vi "readinDioXML.vi"(8 "error in (no error)":errorcluster, 10 "channel_configXML":refnum<class "NativeXML.lvclass">, 11 "deviceDataBase in":refnum<class "deviceDataBase.lvclass">) -> (0 "error out":errorcluster, 2 "device.lvclass out":refnum<class "device.lvclass">, 3 "deviceDataBase out":refnum<class "deviceDataBase.lvclass">)   [LabVIEW 2009, in "Tools.lvlib" / "DatabaseHelpers.lvlib" / "deviceDataBase.lvclass"]
uses:
  deviceDataBase.lvclass
  NativeXML/NativeXML.lvclass
  Database Objects/device/device.lvclass
  Database Objects/device/DigitalDevice/DigitalDevice.lvclass
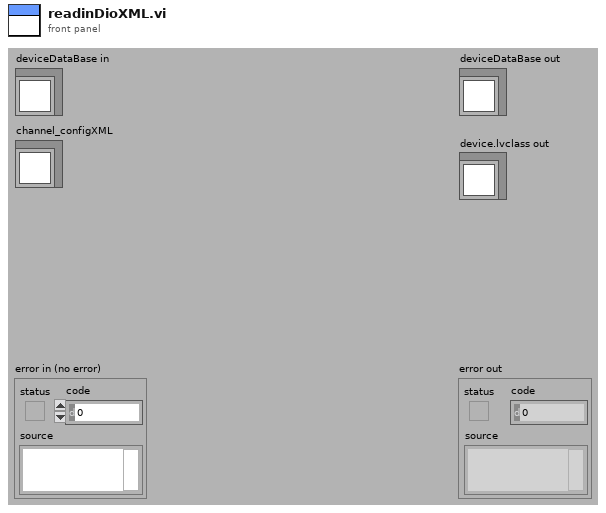
[diagram p1: front panel]
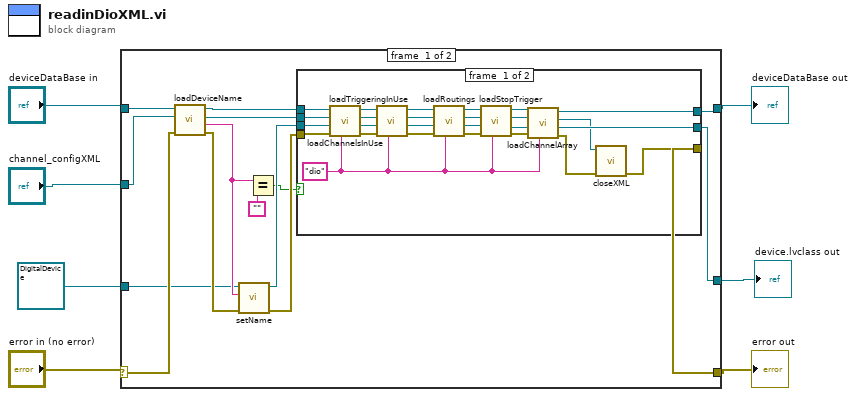
[diagram p0: block diagram]
diagram:
  n1 = case shown="No Error" "error in (no error)" {
    selector: "error in (no error)" -> [w21 w53]
    tunnel: [w9 w53] -> w3
    tunnel: [w14 w52] -> w4
    tunnel: "deviceDataBase in" -> [w22 w52]
    tunnel: "channel_configXML" -> [w20 _]
    tunnel: [w10 _] -> w2
    tunnel: refnum<class "DigitalDevice.lvclass"> refnum ("Tools.lvlib:DatabaseHelpers.lvlib:DigitalDevice.lvclass") -> [w8 _]
    frame #0 {
      n2 = call "loadDeviceName.vi"("error in (no error)"=w21, "NativeXML in"=w20, "deviceDataBase in"=w22) -> ("error out"=w19:errorcluster, "deviceName"=w12:string, "NativeXML out"=w16:refnum<class "NativeXML.lvclass">, "deviceDataBase out"=w18:refnum<class "deviceDataBase.lvclass">)  [unwired: 5 in]
      n3 = call "setName.vi"("error in (no error)"=w19, "name"=w12, "device.lvclass in"=w8) -> ("error out"=w17:errorcluster, "device.lvclass out"=w15:refnum<class "DigitalDevice.lvclass">)  [unwired: 7 in]
      n4 = Equal?(x=w12, y="") -> (x = y?=w11:bool)
      n5 = case shown="False" w11 {
        tunnel: w18 -> [w48 w51]
        tunnel: w17 -> [w47 w49]
        tunnel: w16 -> [w46 _]
        tunnel: w15 -> [w45 w50]
        tunnel: [w23 w49] -> w9
        tunnel: [w40 w50] -> w10
        tunnel: [w39 w51] -> w14
        frame #0 {
          w26 = "dio"
          n6 = call "loadChannelsInUse.vi"("type"=w26, "error in (no error)"=w47, "device.lvclass"=w45, "NativeXML in"=w46, "deviceDataBase in"=w48) -> ("error out"=w44:errorcluster, "device.lvclass out"=w41:refnum<class "device.lvclass">, "NativeXML out"=w42:refnum<class "NativeXML.lvclass">, "deviceDataBase out"=w43:refnum<class "deviceDataBase.lvclass">)  [unwired: 3 in]
          n7 = call "loadTriggeringInUse.vi"("type"=w26, "error in (no error)"=w44, "device.lvclass"=w41, "NativeXML in"=w42, "deviceDataBase in"=w43) -> ("error out"=w35:errorcluster, "device.lvclass out"=w36:refnum<class "device.lvclass">, "NativeXML out"=w37:refnum<class "NativeXML.lvclass">, "deviceDataBase out"=w38:refnum<class "deviceDataBase.lvclass">)  [unwired: 3 in]
          n8 = call "loadRoutings.vi"("type"=w26, "error in (no error)"=w35, "device.lvclass"=w36, "channel_configXML"=w37, "deviceDataBase in"=w38) -> ("error out"=w27:errorcluster, "device.lvclass out"=w31:refnum<class "device.lvclass">, "channel_configXML"=w32:refnum<class "NativeXML.lvclass">, "deviceDataBase out"=w33:refnum<class "deviceDataBase.lvclass">)  [unwired: 3 in]
          n9 = call "loadStopTrigger.vi"("type"=w26, "error in (no error)"=w27, "device.lvclass"=w31, "xml in"=w32, "deviceDataBase in"=w33) -> ("error out"=w28:errorcluster, "device.lvclass out"=w29:refnum<class "device.lvclass">, "xml out"=w30:refnum<class "NativeXML.lvclass">, "deviceDataBase out"=w34:refnum<class "deviceDataBase.lvclass">)  [unwired: 3 in]
          n10 = call "loadChannelArray.vi"("type"=w26, "error in (no error)"=w28, "device.lvclass"=w29, "NativeXML in"=w30, "deviceDataBase in"=w34) -> ("error out"=w25:errorcluster, "device.lvclass out"=w40:refnum<class "device.lvclass">, "NativeXML out"=w24:refnum<class "NativeXML.lvclass">, "deviceDataBase out"=w39:refnum<class "deviceDataBase.lvclass">)  [unwired: 3 in]
          n11 = call "closeXML.vi"("error in (no error)"=w25, "NativeXML in"=w24) -> ("error out"=w23:errorcluster)  [unwired: 9 in]
        }
        frame #1 {
        }
      }
    }
    frame #1 {
    }
  }
  "error out" <- w3
  "deviceDataBase out" <- w4
  "device.lvclass out" <- w2
